vi "TW Post-Project-Copying Process - Stage 3.vi"(8 "error in":errorcluster, 10 "New Subname":string, 11 "Template Project Path":path) -> (0 "error out":errorcluster)   [LabVIEW 2021, in "Plugin Generator.lvlib"]
uses:
  Plugin Generator.lvlib
  <vilib>/CIF Foundation/CIF LabVIEW Scripting/LV Scripting/LV Scripting Utilities.lvlib
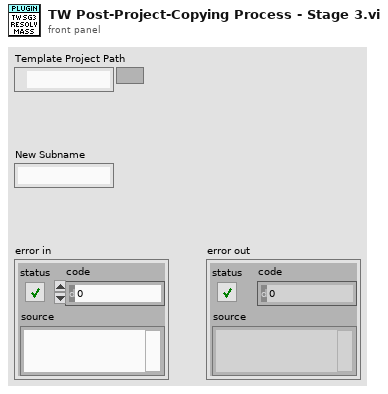
[diagram p1: front panel]
types:
  T1 = typedef "LV Scripting Utilities.lvlib/Target References.ctl" = cluster{"Target Reference":refnum<vi>, "VI References":refnum<vi>[], "Library References":refnum<vi>[], "Build References":refnum<vi>[]}
  T2 = typedef "LV Scripting Utilities.lvlib/Library Map.ctl" = map{string, refnum<vi>}
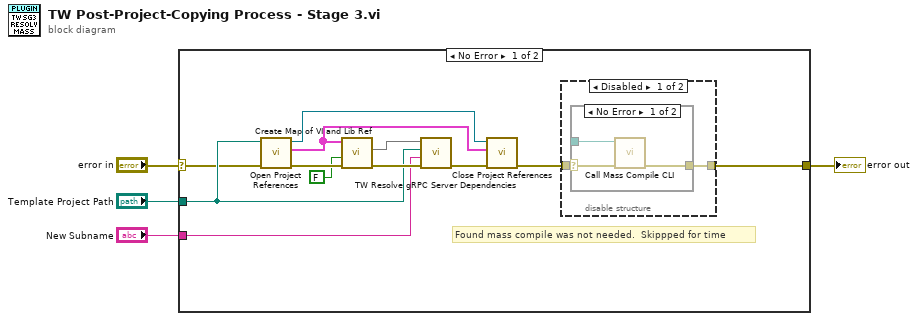
[diagram p0: block diagram]
diagram:
  n1 = case shown="No Error" "error in" {
    selector: "error in" -> [w11 w24]
    tunnel: [w16 w24] -> w4
    tunnel: "New Subname" -> [w13 _]
    tunnel: "Template Project Path" -> [w12 _]
    frame No Error {
      # "Found mass compile was not needed.  Skippped for time"
      n2 = call <vilib>:"Open Project References.vi"("error in"=w11, "Project Path"=w12) -> ("error out"=w10:errorcluster, "VI, Library, and Build References"=w8:T1[], "Project Reference"=w9:refnum<vi>)  [unwired: 7 in]
      n3 = call <vilib>:"Create Map of VI and Lib Ref.vi"("error in"=w10, "RT Target"=FALSE, "VI, Library, and Build References"=w8) -> ("error out"=w14:errorcluster, "Library Map"=w15:T2)  [unwired: 5 in, 2 out]
      n4 = call "TW Resolve gRPC Server Dependencies.vi"("error in"=w14, "New Subname"=w13, "Template Project Path"=w12, "Map - LibRef"=w15) -> ("error out"=w6:errorcluster)  [unwired: 7 in]
      n5 = call <vilib>:"Close Project References.vi"("error in"=w6, "VI, Library, and Build References"=w8, "Project Reference"=w9) -> ("error out"=w5:errorcluster)  [unwired: 8 in]
      n6 = disable-structure shown="Disabled" {
        disable-tunnel: [w18 w23] -> w16
        disable-tunnel: w5 -> [w17 w23]
        frame Disabled {
          n7 = case shown="No Error" w17 {
            selector: w17 -> [w20 w22]
            tunnel: [w19 w22] -> w18
            tunnel: _ -> [w21 _]
            frame No Error {
              n8 = call <vilib>:"Call Mass Compile CLI.vi"("error in"=w20, "Directory"=w21) -> ("error out"=w19:errorcluster)  [unwired: 9 in]
            }
            frame Error {
            }
          }
        }
        frame Enabled {
        }
      }
    }
    frame Error {
    }
  }
  "error out" <- w4
